vi "Appearance Page.vi"() -> ()   [LabVIEW 2020, in "2D Plot.lvclass"]
uses:
  <vilib>/Math Plots/2D Math Plots/2D Plot/2D Plot/2D Plot.lvclass
  <vilib>/Math Plots/2D Math Plots/2D Plot/2D Plot/Typedef/Graph General Property.ctl
  <vilib>/Math Plots/2D Math Plots/2D Plot/Action String/2DMathPlot Ctrl Act Queue.ctl
  <vilib>/Math Plots/2D Math Plots/2D Plot/Action String/2DMathPlot Ctrl Act Cluster.ctl
  <vilib>/Math Plots/2D Math Plots/2D Plot/Action String/2DMathPlot State Class.ctl
  <vilib>/Math Plots/2D Math Plots/2D Plot/2D Plot/Typedef/Dialog State.ctl
  <vilib>/Math Plots/2D Math Plots/2D Plot/2D Plot/Typedef/Temp Graph Property Action.ctl
  <vilib>/Math Plots/2D Math Plots/2D Plot/2D Plot/Typedef/Temp Graph State.ctl
panel:
  in  "Event Registration":refnum<event-registration>
  in  "Control Ref Queue":T1
  out "Graph General Out":T2
  in  "Graph General In":T2
  in  "Legend:Plots Shown":u32=1 caption="Plots shown" min=1
  in  "Autosize Legend":bool caption="Auto size to plot names"
  in  "Cursor Palette Visible":bool caption="Show cursor legend"
  in  "Legend:Visible":bool caption="Show plot legend"
  in  "Scale Legend:Visible":bool caption="Show scale legend"
  in  "Palette:Visible":bool caption="Show graph palette"
  in  "X Scrollbar Visible":bool caption="Show x scroll bar"
  in  "Height":u32 step=1
  in  "Width":u32 step=1
  in  "Enabled State":T3(radio)
  in  "Caption.Visible":bool caption="Caption"
  in  "Caption.Text":string caption="Caption Text"
  in  "Label.Text":string caption="Label Text"
  in  "Label.Visible":bool caption="Label"
  # "Caption"
  # "Label"
  # "Enabled State"
  # "Size"
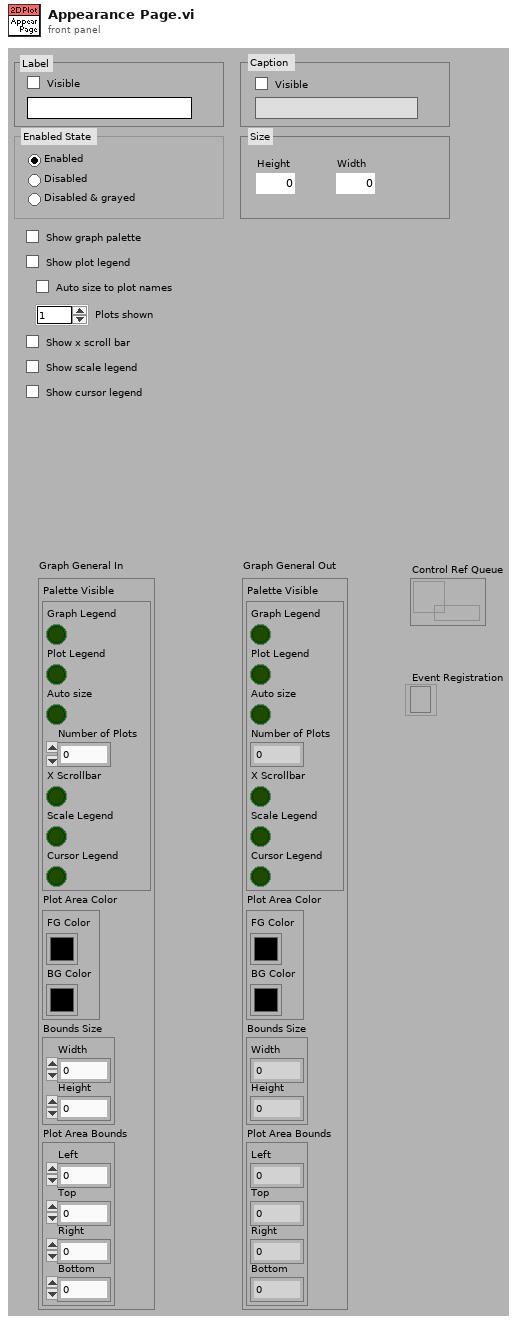
[diagram p1: front panel]
types:
  T1 = typedef "2DMathPlot Ctrl Act Queue.ctl" = refnum<queue>
  T2 = typedef "2D Plot.lvclass/Graph General Property.ctl" = cluster{"Palette Visible":cluster{"Graph Legend":bool, "Plot Legend":bool, "Auto size":bool, "Number of Plots":u32, "X Scrollbar":bool, "Scale Legend":bool, "Cursor Legend":bool}, "Plot Area Color":cluster{"FG Color":u32, "BG Color":u32}, "Bounds Size":cluster{"Width":u32, "Height":u32}, "Plot Area Bounds":cluster{"Left":i16, "Top":i16, "Right":i16, "Bottom":i16}}
  T3 = enum32{"Enabled", "Disabled", "Disabled & grayed", "Multiple Values"}
  T4 = typedef "2D Plot.lvclass/Dialog State.ctl" = enum16{"Initialize", "Read Property", "Write Property", "Idle", "Exit"}
  T5 = typedef "2DMathPlot Ctrl Act Cluster.ctl" = cluster{"Plot Area Ref":refnum<vi>, "Z Axis Ref":refnum<vi>, "Legend Ref":refnum<vi>, "XControl Ref":refnum<vi>, "Facade Ref":refnum<vi>, "Display State Change Class":T6}
  T6 = typedef "2DMathPlot State Class.ctl" = enum16{"Update All (Undo)", "Update General", "Update Appearance", "Update Format", "Update Scale", "Update Marker", "Update Cursor", "None"}
  T7 = typedef "2D Plot.lvclass/Temp Graph State.ctl" = enum16{"Create", "Update Graph", "Update Property Only", "Get Plot Name", "Get Axis Name", "Destory"}
  T8 = typedef "2D Plot.lvclass/Temp Graph Property Action.ctl" = enum16{"Appearance Property", "Format Property", "Plots Property", "Scales Property"}
  T9 = enum8{"Enabled", "Disabled", "Disabled and Grayed Out"}
  T10 = cluster{"Left":i16, "Top":i16, "Right":i16, "Bottom":i16}
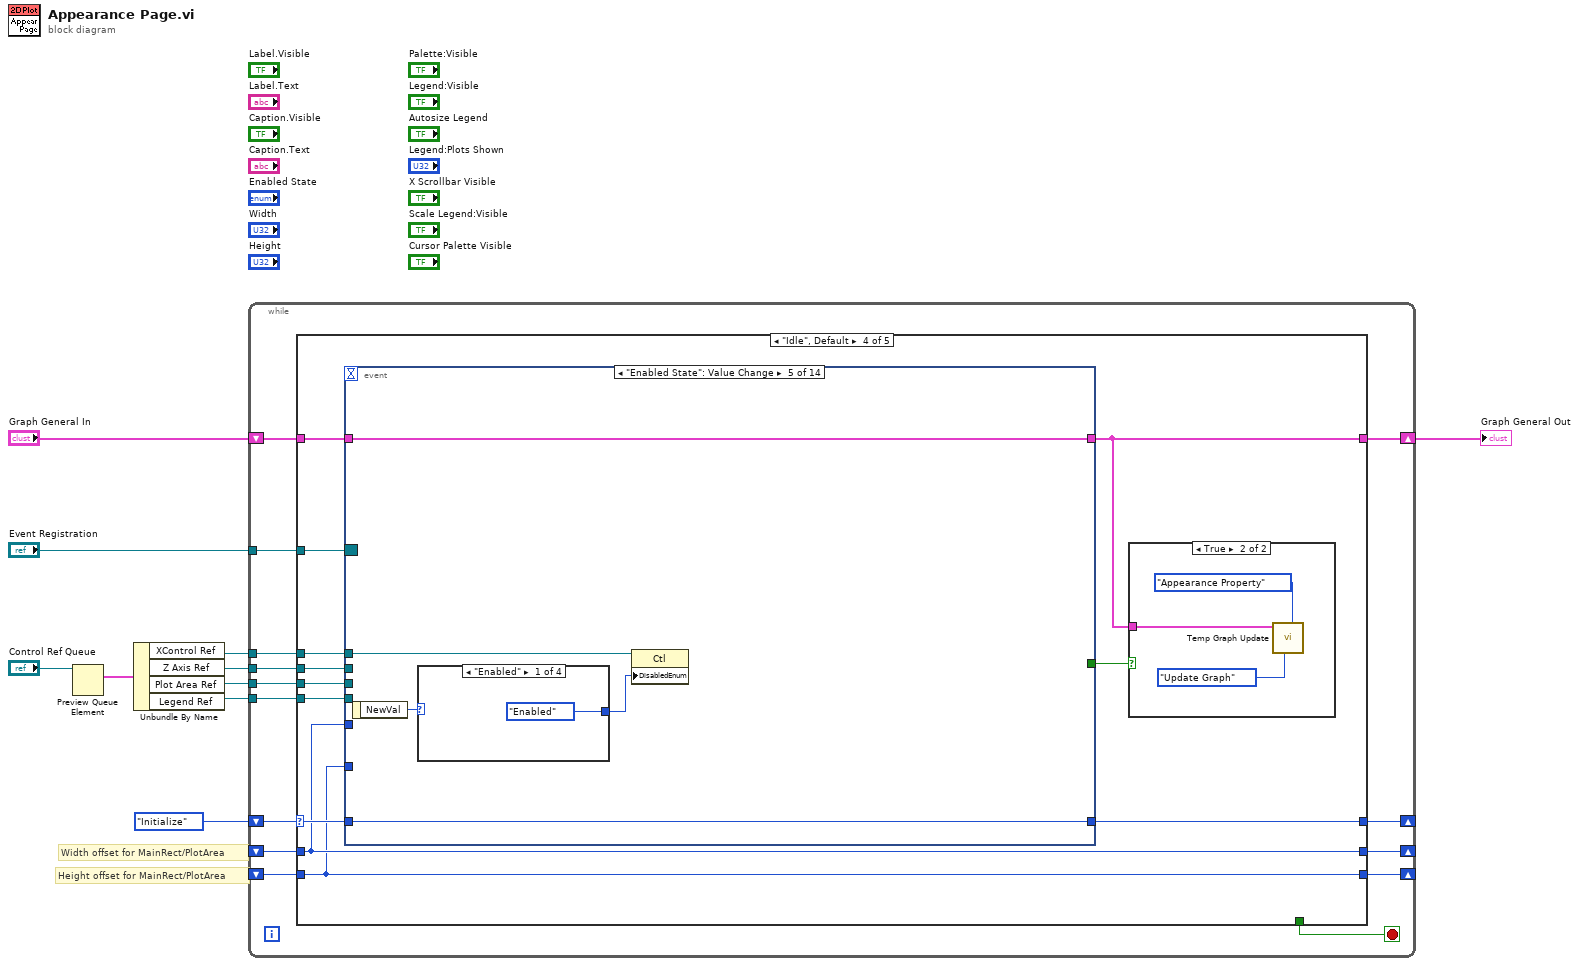
[diagram p0: block diagram]
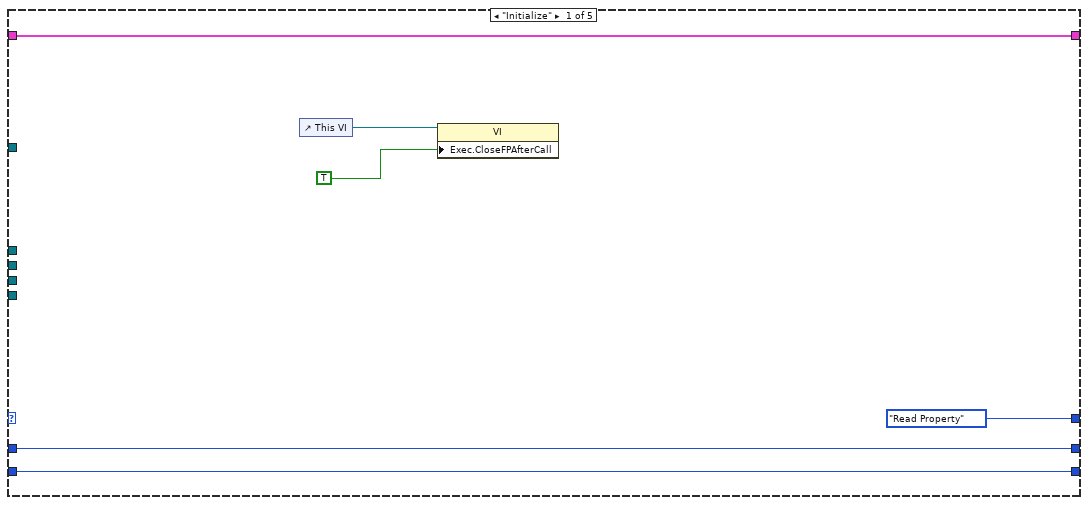
[diagram p2: hidden frame]
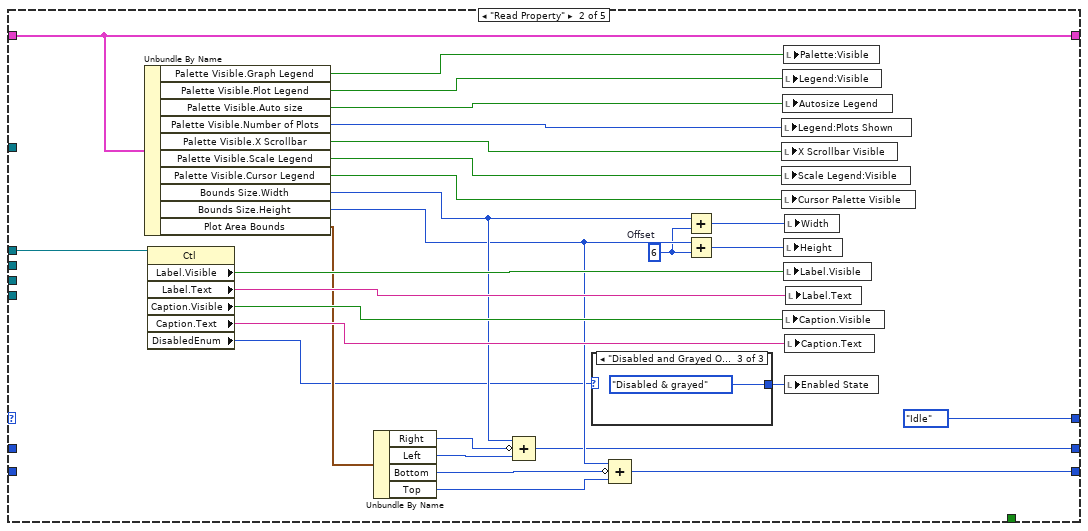
[diagram p3: hidden frame]
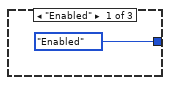
[diagram p4: hidden frame]
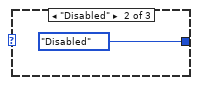
[diagram p5: hidden frame]
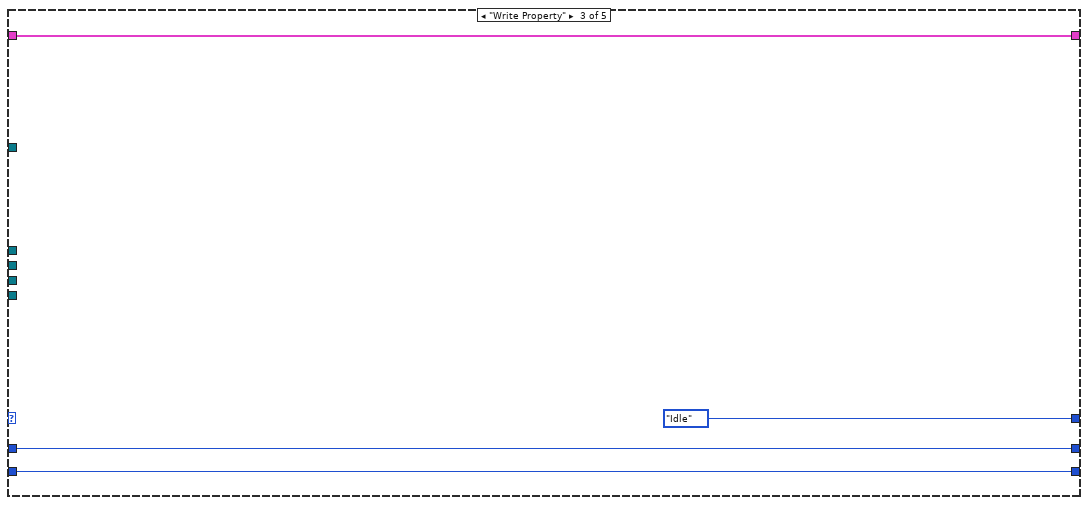
[diagram p6: hidden frame]
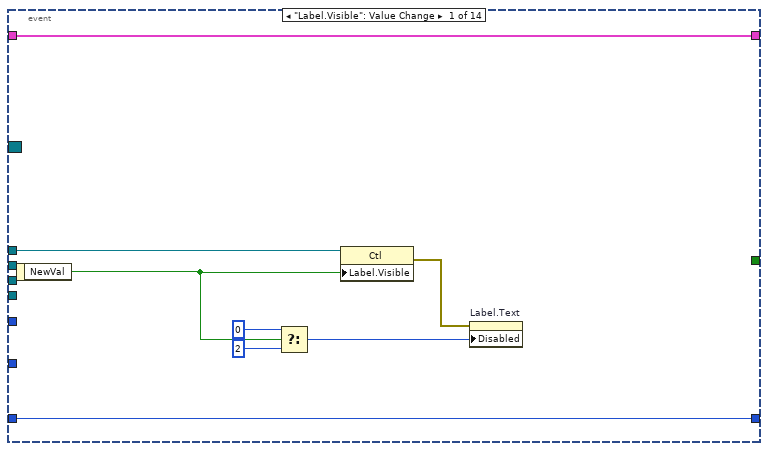
[diagram p8: hidden frame]
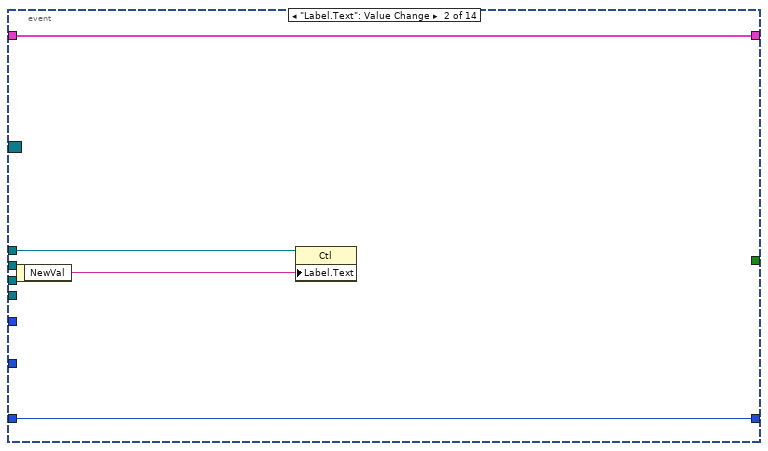
[diagram p9: hidden frame]
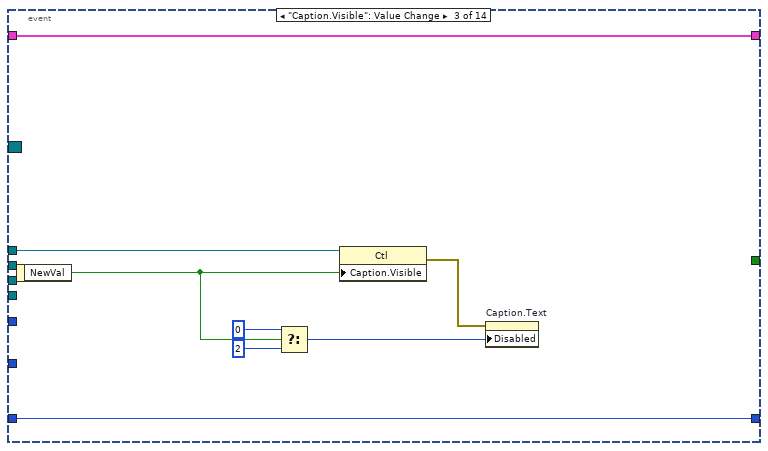
[diagram p10: hidden frame]
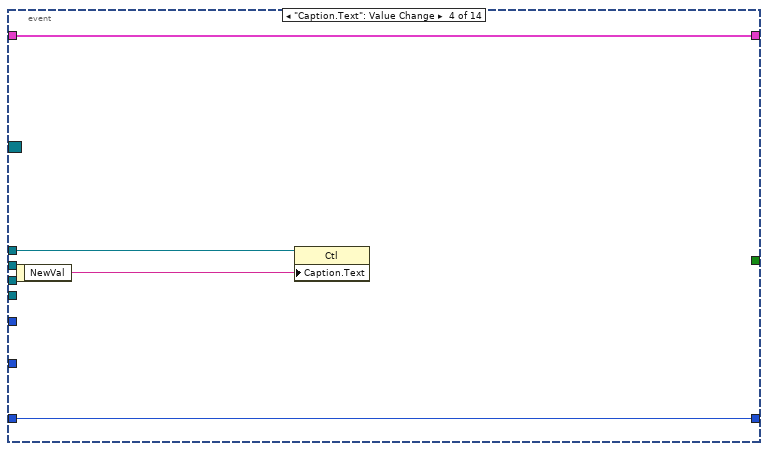
[diagram p11: hidden frame]
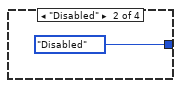
[diagram p12: hidden frame]
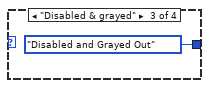
[diagram p13: hidden frame]
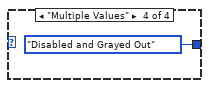
[diagram p14: hidden frame]
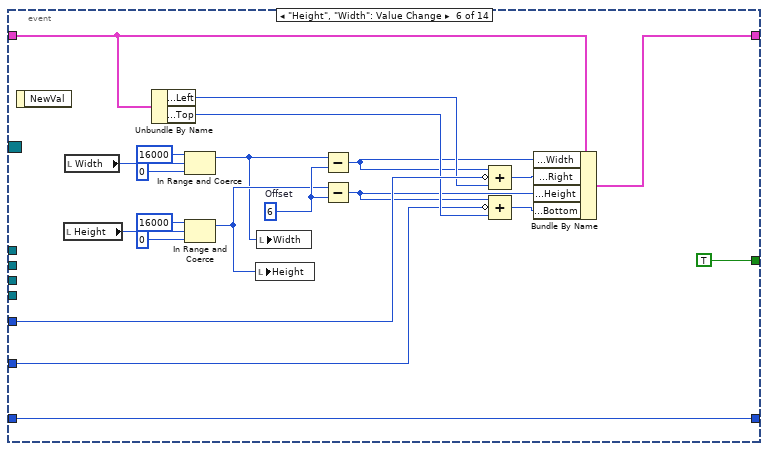
[diagram p15: hidden frame]
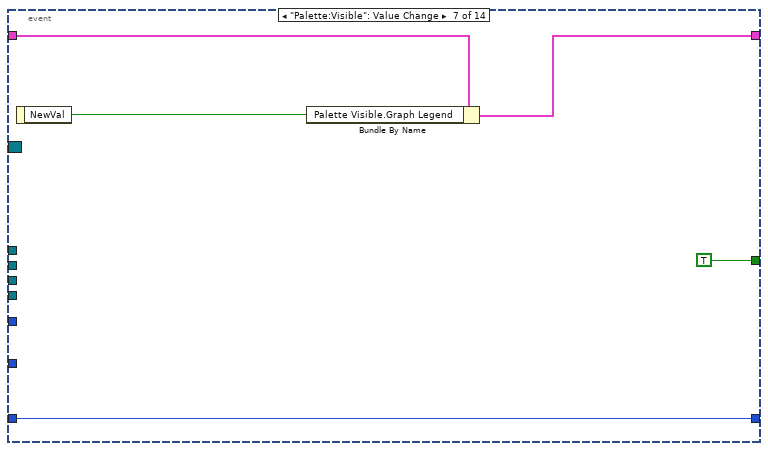
[diagram p16: hidden frame]
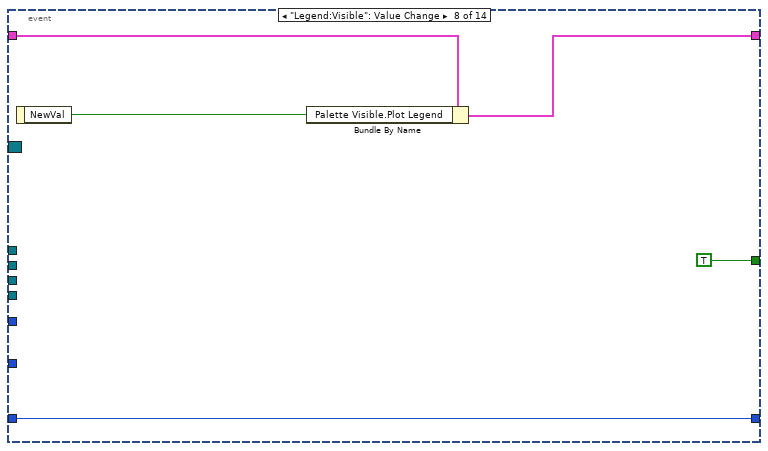
[diagram p17: hidden frame]
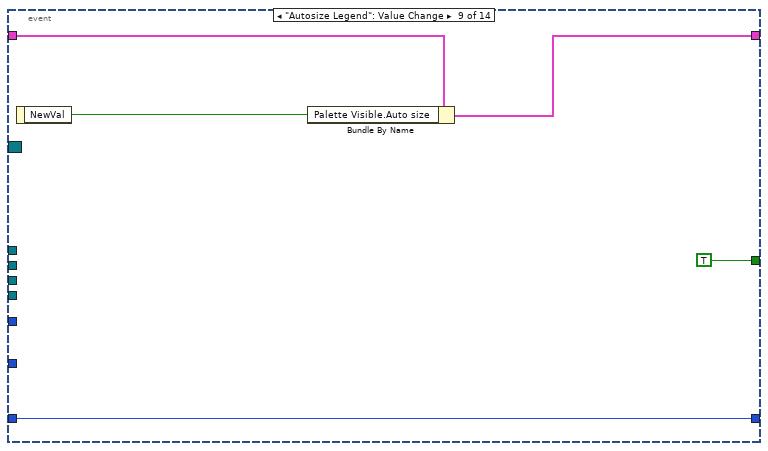
[diagram p18: hidden frame]
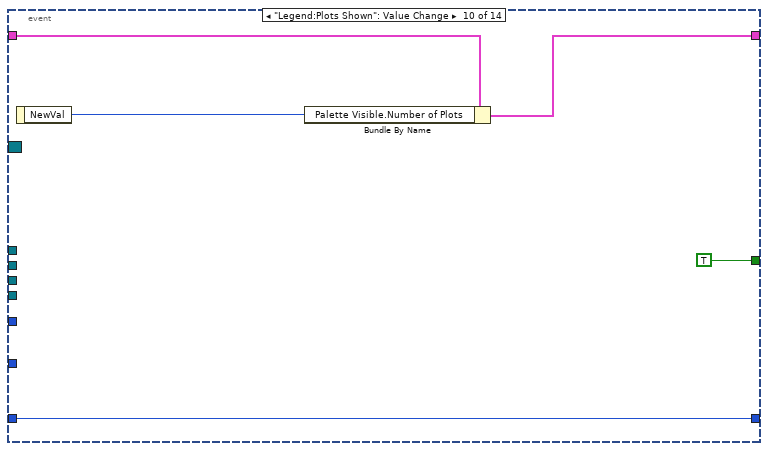
[diagram p19: hidden frame]
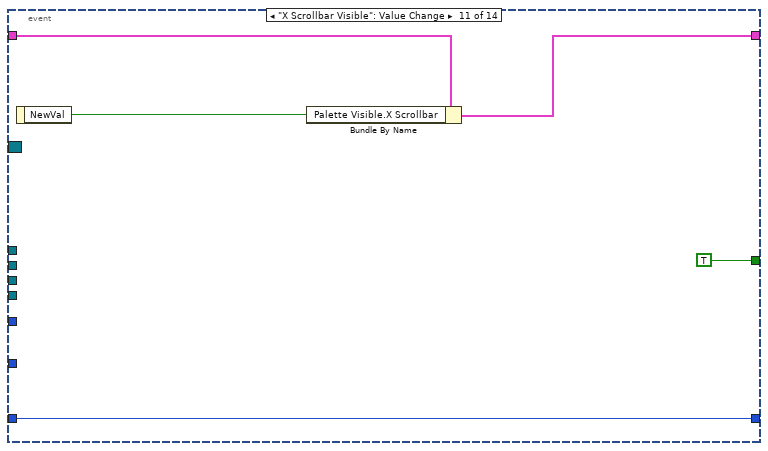
[diagram p20: hidden frame]
diagram:
  # "Height offset for MainRect/PlotArea"
  # "Width offset for MainRect/PlotArea"
  n1 = Preview Queue Element(queue="Control Ref Queue") -> (element=w2:T5)  [unwired: 1 in, 4 out]
  n2 = Unbundle By Name(w2) -> ("XControl Ref"=w6:refnum<vi>, "Z Axis Ref"=w5:refnum<vi>, "Plot Area Ref"=w4:refnum<vi>, "Legend Ref"=w1:refnum<vi>)
  n3 = while {
    shift-right: [w22] -> _
    shift-left: Dialog_State."Initialize" ("Enum") -> [w24]
    shift-right: [w21] -> w9
    shift-left: "Graph General In" -> [w20]
    tunnel: w6 -> [w19]
    tunnel: w5 -> [w18]
    tunnel: w4 -> [w17]
    tunnel: "Event Registration" -> [w16]
    shift-right: [w15] -> _
    shift-left: _ -> [w13]
    shift-right: [w14] -> _
    shift-left: _ -> [w12]
    tunnel: w1 -> [w11]
    stop <- w23 stop-if-true
    n4 = case shown="\"Idle\", Default" w24 {
      selector: w24 -> [_ _ _ w71 w175]
      tunnel: [_ _ _ _ TRUE] -> w23
      tunnel: [Dialog_State."Read Property" ("Enum") Dialog_State."Idle" ("Enum") Dialog_State."Idle" ("Enum") w72 w175] -> w22
      tunnel: [w27 w45 w64 w66 w174] -> w21
      tunnel: w20 -> [w27 w45 w64 w77 w174]
      tunnel: w19 -> [_ w50 _ w76 _]
      tunnel: w18 -> [_ _ _ w75 _]
      tunnel: w17 -> [_ _ _ w74 _]
      tunnel: w16 -> [_ _ _ w73 _]
      tunnel: [w26 w36 w63 w69 w173] -> w15
      tunnel: [w25 w37 w62 w68 w172] -> w14
      tunnel: w13 -> [w26 _ w63 w69 w173]
      tunnel: w12 -> [w25 _ w62 w68 w172]
      tunnel: w11 -> [_ _ _ w67 _]
      frame "Initialize" {
        n5 = control-ref of="This VI"() -> (w29:refnum<vi>)
        n6 = property class="VI"(reference=w29, "Exec.CloseFPAfterCall"=TRUE ("Execution:Close After Call")) -> ()  [unwired: 1 in, 2 out]
      }
      frame "Read Property" {
        w33 = u32 6  # Offset
        n7 = Unbundle By Name(w45) -> ("Palette Visible.Graph Legend"=w57:bool, "Palette Visible.Plot Legend"=w56:bool, "Palette Visible.Auto size"=w55:bool, "Palette Visible.Number of Plots"=w54:u32, "Palette Visible.X Scrollbar"=w53:bool, "Palette Visible.Scale Legend"=w52:bool, "Palette Visible.Cursor Legend"=w51:bool, "Bounds Size.Width"=w43:u32, "Bounds Size.Height"=w40:u32, "Plot Area Bounds"=w44:T10)
        n8 = property class="Ctl"(reference=w50) -> ("Label.Visible"=w49:bool, "Label.Text"=w48:string, "Caption.Visible"=w47:bool, "Caption.Text"=w46:string, "DisabledEnum"=w32:T9)  [unwired: 1 in, 2 out]
        n9 = Unbundle By Name(w44) -> ("Right"=w42:i16, "Left"=w41:i16, "Bottom"=w39:i16, "Top"=w38:i16)
        n10 = Compound Arithmetic op=ADD(w43, invert w42, w41) -> (w36:u32)
        n11 = case shown="\"Disabled and Grayed Out\"" w32 {
          tunnel: [T3."Enabled" ("Enabled State") T3."Disabled" ("Enabled State") T3."Disabled & grayed" ("Enabled State")] -> w31
          frame "Enabled" {
          }
          frame "Disabled" {
          }
          frame "Disabled and Grayed Out" {
          }
        }
        n12 = Compound Arithmetic op=ADD(w40, invert w39, w38) -> (w37:u32)
        n13 = Add(x=w43, y=w33) -> (x+y=w35:u32)
        n14 = Add(x=w40, y=w33) -> (x+y=w34:u32)
        n15 = local write "Legend:Plots Shown"(w54) -> ()
        n16 = local write "X Scrollbar Visible"(w53) -> ()
        n17 = local write "Scale Legend:Visible"(w52) -> ()
        n18 = local write "Cursor Palette Visible"(w51) -> ()
        n19 = local write "Legend:Visible"(w56) -> ()
        n20 = local write "Autosize Legend"(w55) -> ()
        n21 = local write "Caption.Visible"(w47) -> ()
        n22 = local write "Palette:Visible"(w57) -> ()
        n23 = local write "Height"(w34) -> ()
        n24 = local write "Label.Visible"(w49) -> ()
        n25 = local write "Width"(w35) -> ()
        n26 = local write "Caption.Text"(w46) -> ()
        n27 = local write "Enabled State"(w31) -> ()
        n28 = local write "Label.Text"(w48) -> ()
      }
      frame "Write Property" {
      }
      frame "Idle", Default {
        n29 = event shown="[4] \"Enabled State\": Value Change" {
          selector: w73 -> [_ _ _ _ _ _ _ _ _ _ _ _ _ _]
          dyn-events: _ -> [_ _ _ _ _ _ _ _ _ _ _ _ _ _]
          timeout: _ -> [_ _ _ _ _ _ _ _ _ _ _ _ _ _]
          tunnel: w77 -> [w88 w90 w100 w102 w108 w131 w139 w144 w149 w154 w159 w164 w169 w171]
          tunnel: [w88 w90 w100 w102 w108 w133 w138 w143 w148 w153 w158 w163 w168 w171] -> w66
          tunnel: w76 -> [w87 w92 w99 w104 w109 _ _ _ _ _ _ _ _ _]
          tunnel: w75 -> [_ _ _ _ _ _ _ _ _ _ _ _ _ _]
          tunnel: w74 -> [_ _ _ _ _ _ _ _ _ _ _ _ _ _]
          tunnel: [w81 w89 w93 w101 w107 w134 w136 w141 w146 w151 w156 w161 w166 Dialog_State."Exit" ("Enum")] -> w72
          tunnel: w71 -> [w81 w89 w93 w101 w107 w134 w136 w141 w146 w151 w156 w161 w166 _]
          tunnel: [_ _ _ _ _ TRUE TRUE TRUE TRUE TRUE TRUE TRUE TRUE _] -> w70
          tunnel: w69 -> [_ _ _ _ _ w130 _ _ _ _ _ _ _ _]
          tunnel: w68 -> [_ _ _ _ _ w125 _ _ _ _ _ _ _ _]
          tunnel: w67 -> [_ _ _ _ _ _ _ _ _ _ _ _ _ _]
          event "Label.Visible": Value Change {
            n30 = event-data() -> ("NewVal"=w86:bool)  [unwired: 1 out]
            n31 = Select(t=u8 0 ("Disabled"), s=w86, f=u8 2 ("Disabled")) -> (s? t:f=w83:u8)
            n32 = property class="Ctl"(reference=w87, "Label.Visible"=w86) -> (error out=w82:errorcluster)  [unwired: 1 in, 1 out]
            n33 = property on="Label.Text" class="Str"(error in=w82, "Disabled"=w83) -> ()  [unwired: 1 in, 2 out]
          }
          event "Label.Text": Value Change {
            n34 = event-data() -> ("NewVal"=w91:string)  [unwired: 1 out]
            n35 = property class="Ctl"(reference=w92, "Label.Text"=w91) -> ()  [unwired: 1 in, 2 out]
          }
          event "Caption.Visible": Value Change {
            n36 = event-data() -> ("NewVal"=w98:bool)  [unwired: 1 out]
            n37 = Select(t=u8 0 ("Disabled"), s=w98, f=u8 2 ("Disabled")) -> (s? t:f=w95:u8)
            n38 = property class="Ctl"(reference=w99, "Caption.Visible"=w98) -> (error out=w94:errorcluster)  [unwired: 1 in, 1 out]
            n39 = property on="Caption.Text" class="Str"(error in=w94, "Disabled"=w95) -> ()  [unwired: 1 in, 2 out]
          }
          event "Caption.Text": Value Change {
            n40 = event-data() -> ("NewVal"=w103:string)  [unwired: 1 out]
            n41 = property class="Ctl"(reference=w104, "Caption.Text"=w103) -> ()  [unwired: 1 in, 2 out]
          }
          event "Enabled State": Value Change {
            n42 = event-data() -> ("NewVal"=w106:T3)  [unwired: 1 out]
            n43 = case shown="\"Enabled\"" w106 {
              tunnel: [T9."Enabled" ("Disabled") T9."Disabled" ("Disabled") T9."Disabled and Grayed Out" ("Disabled") T9."Disabled and Grayed Out" ("Disabled")] -> w105
              frame "Enabled" {
              }
              frame "Disabled" {
              }
              frame "Disabled & grayed" {
              }
              frame "Multiple Values" {
              }
            }
            n44 = property class="Ctl"(reference=w109, "DisabledEnum"=w105) -> ()  [unwired: 1 in, 2 out]
          }
          event "Height", "Width": Value Change {
            w124 = u32 6  # Offset
            n45 = event-data() -> ()  [unwired: 2 out]
            n46 = local read "Height"() -> (w119:u32)
            n47 = local read "Width"() -> (w116:u32)
            n48 = Unbundle By Name(w131) -> ("Plot Area Bounds.Left"=w129:i16, "Plot Area Bounds.Top"=w128:i16)
            n49 = In Range and Coerce(upper limit=u32 16000, x=w116, lower limit=u32 0) -> (coerced(x)=w114:u32)  [unwired: 1 out]
            n50 = In Range and Coerce(upper limit=u32 16000, x=w119, lower limit=u32 0) -> (coerced(x)=w115:u32)  [unwired: 1 out]
            n51 = local write "Height"(w115) -> ()
            n52 = local write "Width"(w114) -> ()
            n53 = Subtract(x=w114, y=w124) -> (x-y=w122:u32)
            n54 = Subtract(x=w115, y=w124) -> (x-y=w123:u32)
            n55 = Compound Arithmetic op=ADD(w122, invert w130, w129) -> (w126:u32)
            n56 = Compound Arithmetic op=ADD(w123, invert w125, w128) -> (w127:u32)
            n57 = Bundle By Name(cluster=w131, "Bounds Size.Width"=w122, "Plot Area Bounds.Right"=w126, "Bounds Size.Height"=w123, "Plot Area Bounds.Bottom"=w127) -> (w133:T2)
          }
          event "Palette:Visible": Value Change {
            n58 = event-data() -> ("NewVal"=w137:bool)  [unwired: 1 out]
            n59 = Bundle By Name(cluster=w139, "Palette Visible.Graph Legend"=w137) -> (w138:T2)
          }
          event "Legend:Visible": Value Change {
            n60 = event-data() -> ("NewVal"=w142:bool)  [unwired: 1 out]
            n61 = Bundle By Name(cluster=w144, "Palette Visible.Plot Legend"=w142) -> (w143:T2)
          }
          event "Autosize Legend": Value Change {
            n62 = event-data() -> ("NewVal"=w147:bool)  [unwired: 1 out]
            n63 = Bundle By Name(cluster=w149, "Palette Visible.Auto size"=w147) -> (w148:T2)
          }
          event "Legend:Plots Shown": Value Change {
            n64 = event-data() -> ("NewVal"=w152:u32)  [unwired: 1 out]
            n65 = Bundle By Name(cluster=w154, "Palette Visible.Number of Plots"=w152) -> (w153:T2)
          }
          event "X Scrollbar Visible": Value Change {
            n66 = event-data() -> ("NewVal"=w157:bool)  [unwired: 1 out]
            n67 = Bundle By Name(cluster=w159, "Palette Visible.X Scrollbar"=w157) -> (w158:T2)
          }
          event "Scale Legend:Visible": Value Change {
            n68 = event-data() -> ("NewVal"=w162:bool)  [unwired: 1 out]
            n69 = Bundle By Name(cluster=w164, "Palette Visible.Scale Legend"=w162) -> (w163:T2)
          }
          event "Cursor Palette Visible": Value Change {
            n70 = event-data() -> ("NewVal"=w167:bool)  [unwired: 1 out]
            n71 = Bundle By Name(cluster=w169, "Palette Visible.Cursor Legend"=w167) -> (w168:T2)
          }
          event User Event {
            n72 = event-data() -> ()  [unwired: 6 out]
          }
        }
        n73 = case shown="True" w70 {
          tunnel: w66 -> [_ w80]
          frame False {
          }
          frame True {
            n74 = call <vilib>:"Temp Graph Update.vi"("Property Name"=Temp_Graph_Property_Action."Appearance Property", "State"=Temp_Graph_State."Update Graph", "Property In"=w80) -> ()  [unwired: 2 in, 7 out]
          }
        }
      }
      frame "Exit" {
      }
    }
  }
  "Graph General Out" <- w9
